vi "get_enum_value.vi"(7 "Attribute":T1={"Identifier"="", "Descriptive name"="", "Data Type"=enum."Integer 32", "Command"="", "Access"=2, "Range Table"="", "Read Callback"="", "Write Callback"="", "Range Callback"="", "Check Callback"="", "Rngtable Callback"="", "Coerce Callback"="", "Supported Models"="", "Instrument Options"="", "Repeated Capabilities"="", "Check Status Callback"="", "Index"=0, "Flag: OPC Wait"=FALSE, "Flag: Dont check status"=FALSE, "Flag: Cache Only"=FALSE} {"Access" items=["Read Only", "Write Only", "Read/Write"]}, 8 "error in":errorcluster, 10 "String Value":string, 11 "VISA resource name":refnum<visa-resource-name>) -> (0 "error out":errorcluster, 2 "I32 output":i32, 3 "VISA resource name out":refnum<visa-resource-name>)   [LabVIEW 2014, in "rszvl_rsidr_core.lvlib"]
uses:
  rszvl_rsidr_core.lvlib
  type_Attribute.ctl
  type_Attribute_Data_Type.ctl
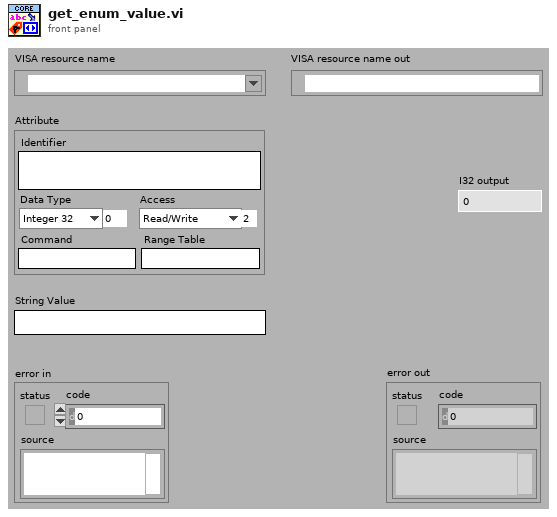
[diagram p1: front panel]
types:
  T1 = typedef "rszvl_rsidr_core.lvlib/type_Attribute.ctl" = cluster{"Identifier":string, "Descriptive name":string, "Data Type":T2, "Command":string, "Access":u16, "Range Table":string, "Read Callback":string, "Write Callback":string, "Range Callback":string, "Check Callback":string, "Rngtable Callback":string, "Coerce Callback":string, "Supported Models":string, "Instrument Options":string, "Repeated Capabilities":string, "Check Status Callback":string, "Index":i32, "Flag: OPC Wait":bool, "Flag: Dont check status":bool, "Flag: Cache Only":bool}
  T2 = typedef "rszvl_rsidr_core.lvlib/type_Attribute_Data_Type.ctl" = enum16{"Integer 32", "Double", "String", "Boolean", "None", "Integer 64"}
  T3 = enum16{"Initialize", "Check", "Get Numeric Value", "Get Default Value"}
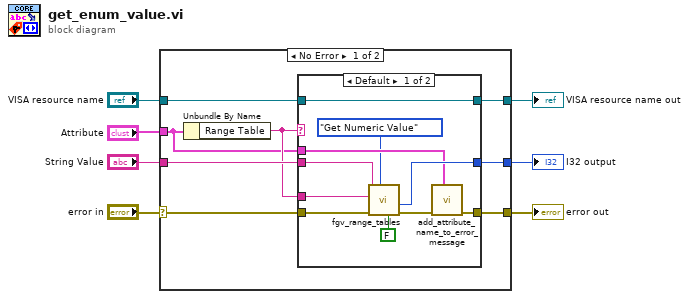
[diagram p0: block diagram]
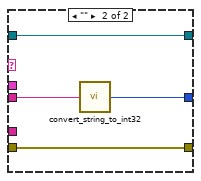
[diagram p2: hidden frame]
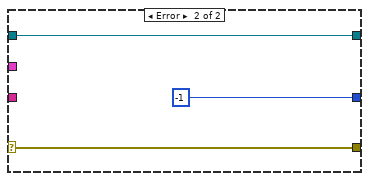
[diagram p3: hidden frame]
diagram:
  n1 = case shown="No Error" "error in" {
    selector: "error in" -> [w13 w32]
    tunnel: [w15 w32] -> w7
    tunnel: [w14 -1] -> w5
    tunnel: "VISA resource name" -> [w12 w30]
    tunnel: [w11 w30] -> w3
    tunnel: "Attribute" -> [w8 _]
    tunnel: "String Value" -> [w10 _]
    frame No Error {
      n2 = Unbundle By Name(w8) -> ("Range Table"=w9:string)
      n3 = case shown="Default" w9 {
        tunnel: w13 -> [w25 w29]
        tunnel: [w19 w29] -> w15
        tunnel: w9 -> [w24 _]
        tunnel: [w22 w26] -> w14
        tunnel: w10 -> [w23 w27]
        tunnel: w12 -> [w21 w28]
        tunnel: [w21 w28] -> w11
        tunnel: w8 -> [w18 _]
        frame Default {
          n4 = call "fgv_range_tables.vi"("Range Checking"=FALSE ("Range Checking Disabled"), "Operation"=T3."Get Numeric Value", "error in"=w25, "Range Table ID in"=w24, "Query String in (\"\")"=w23) -> ("error out"=w17:errorcluster, "Numeric I32 Value out"=w22:i32)  [unwired: 3 in, 2 out]
          n5 = call "add_attribute_name_to_error_message.vi"("Attribute"=w18, "error in"=w17) -> ("error out"=w19:errorcluster)  [unwired: 8 in, 1 out]
        }
        frame "" {
          n6 = call "convert_string_to_int32.vi"("String in"=w27) -> ("int32 value out"=w26:i32)  [unwired: 4 in]
        }
      }
    }
    frame Error {
    }
  }
  "VISA resource name out" <- w3
  "error out" <- w7
  "I32 output" <- w5
